vi "Blynk LCD.vi"(4 "coord_y":string, 6 "coord_x":string, 8 "error in":errorcluster, 9 "value":string, 10 "pin":string, 11 "connection":refnum<k5>) -> (0 "error out":errorcluster, 3 "connection out":refnum<k5>)   [LabVIEW 2014]
uses:
  utilities/MsgType.ctl
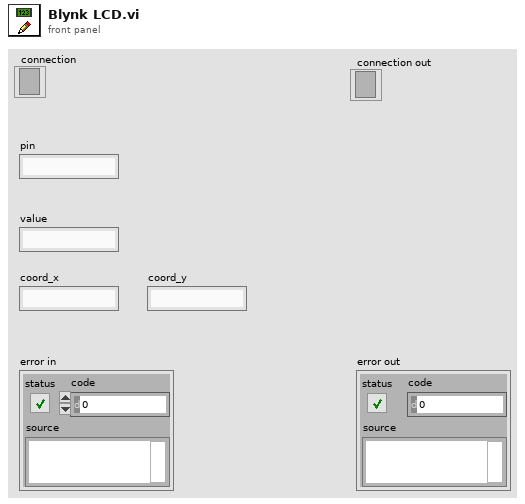
[diagram p1: front panel]
types:
  T1 = typedef "MsgType.ctl" = enum8{"RSP", "REGISTER", "LOGIN", "SAVE_PROF", "LOAD_PROF", "GET_TOKEN", "PING", "ACTIVATE", "DEACTIVATE", "REFRESH", "UNDEFINED0", "UNDEFINED1", "TWEET", "EMAIL", "NOTIFY", "BRIDGE", "UNDEFINED2", "UNDEFINED3", "UNDEFINED4", "UNDEFINED5", "HW"}
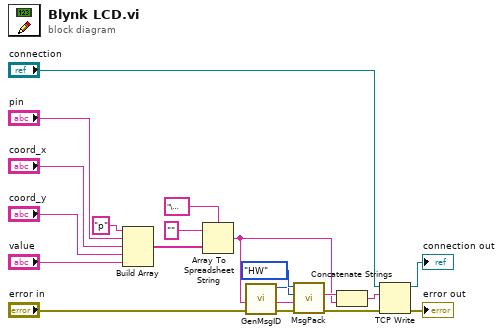
[diagram p0: block diagram]
diagram:
  n1 = Build Array("p" ("format string"), "pin", "coord_x", "coord_y", "value") -> (w10:string[])
  n2 = Array To Spreadsheet String(delimiter (Tab)="\u0000", array=w10, 3:"" ("format string")) -> (spreadsheet string=w15:string)
  n3 = call "GenMsgID.vi"() -> ("MsgID"=w4:u16)  [unwired: 10 in, 1 out]
  n4 = call "MsgPack.vi"("error in"="error in", "msg"=w15, "msg_id"=w4, "msg_type"=MsgType."HW") -> ("error out"=w13:errorcluster, "msg_data"=w16:string)  [unwired: 6 in]
  n5 = Concatenate Strings(w16, w15) -> (w14:string)
  n6 = TCP Write(connection ID="connection", data in=w14, error in (no error)=w13) -> (connection ID out=→"connection out":refnum<k5>, error out=→"error out":errorcluster)  [unwired: 1 in, 1 out]
